vi "plan_to_coordinates.vi"(3 "error in (no error)":errorcluster, 5 "Plan GCode":string) -> (0 "error out":errorcluster, 2 "XY Graph":cluster{"X":dbl, "Y":dbl}[](array[cluster]))   [LabVIEW 2020]
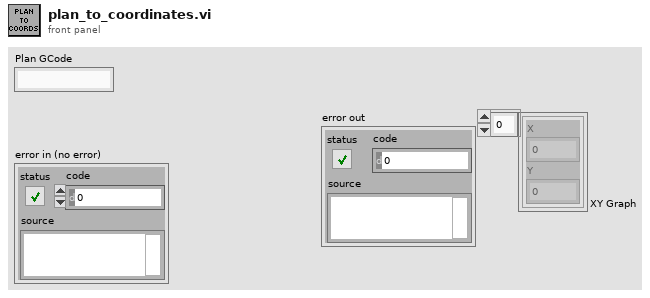
[diagram p1: front panel]
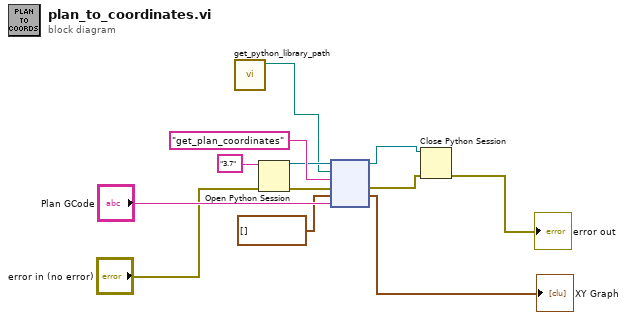
[diagram p0: block diagram]
diagram:
  n1 = call "get_python_library_path.vi"() -> ("Python library path"=w3:path)  [unwired: 11 in]
  n2 = Open Python Session(python version="3.7" ("Python version"), 3:"error in (no error)") -> (session out=w5:refnum<k35>, error out=w7:errorcluster)  [unwired: 1 in]
  n3 = node(w5, w3, "get_plan_coordinates" ("function name"), w7, cluster{"X":dbl, "Y":dbl}[] [] ("XY Graph"), "Plan GCode") -> (w10:refnum<k35>, w11:errorcluster, →"XY Graph":cluster{"X":dbl, "Y":dbl}[])  [unwired: 1 in, 2 out]
  n4 = Close Python Session(session in=w10, error in=w11) -> (11:→"error out":errorcluster)
